vi "CTRE_CANifier_ConfigClearPositionOnQuadIdx.vi"(6 "timeoutMs":i32, 8 "error in":errorcluster, 10 "clearPositionOnQuadIdx":bool=TRUE, 11 "CANifierDevRef":T1) -> (0 "error out":errorcluster, 3 "CANifierDevRef":T1)   [LabVIEW 2020]
uses:
  <vilib>/Rock Robotics/WPI/ThirdParty/Phoenix-LabVIEW/CANifier/CTRE_CANifier_DeviceRef.ctl
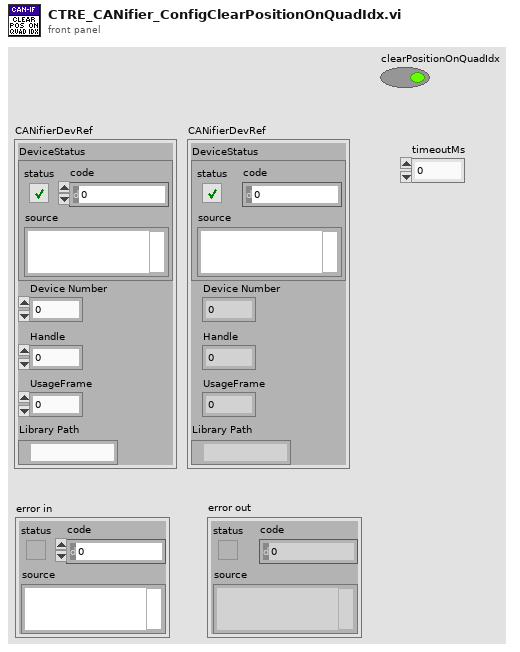
[diagram p1: front panel]
types:
  T1 = typedef "CTRE_CANifier_DeviceRef.ctl" = cluster{"DeviceStatus":errorcluster, "Device Number":u8, "Handle":u64, "UsageFrame":u32, "Library Path":path}
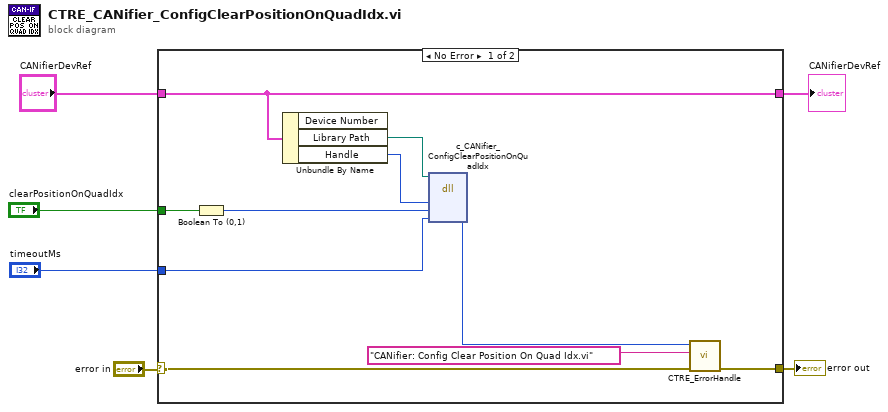
[diagram p0: block diagram]
diagram:
  n1 = case shown="No Error" "error in" {
    selector: "error in" -> [w8 w18]
    tunnel: [w9 w18] -> w5
    tunnel: "CANifierDevRef" -> [w16 w17]
    tunnel: [w16 w17] -> w3
    tunnel: "clearPositionOnQuadIdx" -> [w12 _]
    tunnel: "timeoutMs" -> [w7 _]
    frame No Error {
      n2 = Boolean To (0,1)(Boolean=w12) -> (0, 1=w11:i16)
      n3 = Unbundle By Name(w16) -> ("Library Path"=w15:path, "Handle"=w14:u64)  [unwired: 1 out]
      n4 = dll-call lib="?" fn="c_CANifier_ConfigClearPositionOnQuadIdx"(path in=w15, "handle"=w14, "clearPositionOnQuadIdx"=w11, "timeoutMs"=w7) -> ("CTR_Code"=w13:i8)  [unwired: 5 in, 2 out]
      n5 = call <vilib>:"CTRE_ErrorHandle.vi"("error in"=w8, "origin"="CANifier: Config Clear Position On Quad Idx.vi", "code"=w13) -> ("error out"=w9:errorcluster)  [unwired: 8 in]
    }
    frame Error {
    }
  }
  "error out" <- w5
  "CANifierDevRef" <- w3
